vi "ziImpedance.vi"(9 "Eq Model":T1, 10 "Z (Ohm)":cdb[](array[numeric]) format="%_5p", 11 "Frequency (Hz)":dbl[](array[numeric]) format="%_6p") -> (2 "Labels and Units":string[][](array[string]), 3 "Values":dbl[][](array[numeric]))   [LabVIEW 2009, in "Zurich Instruments LabOne.lvlib"]
doc: "Calculate effective resistance, admittance and equivalen R||C circuit parameters for a DUT measured with an HF2 and an HF2CA.\n\n<B>Stimulation Amplitude (V)</B> (complex) in 4-point mode is the complex voltage amplitude measured accross the DUT (the user needs to account for Vrms to Vamplitude conversion by multiplying with sqrt(2)), in 2-point mode is the voltage amplitude applied to the DUT.\n<B>Measured (Vrms)</B> (complex) the measurement from HF2Camp.\n<B>Rci, Cci</B> Parasitic impedance between Z and preamp to gnd."
uses:
  <instrlib>/Zurich Instruments LabOne/Zurich Instruments LabOne.lvlib
  <instrlib>/Zurich Instruments LabOne/Public/Utility/Impedance/ziTypeImpedanceEqCircModel.ctl
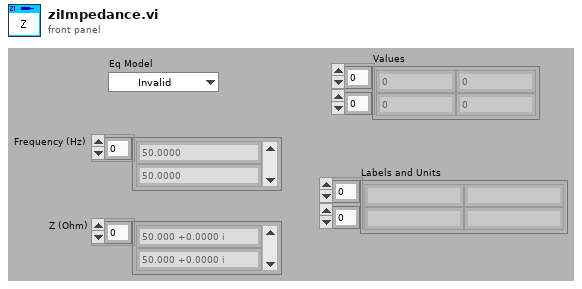
[diagram p1: front panel]
types:
  T1 = typedef "Zurich Instruments LabOne.lvlib/ziTypeImpedanceEqCircModel.ctl" = enum16{"Invalid", "|Z|, Phi", "R||C", "R||L", "R*C", "D*C", "R*L", "ReZ, ImZ", "G, B"}
  T2 = cluster{"label1":string, "label 2":string, "unit1":string, "unit2":string}[]
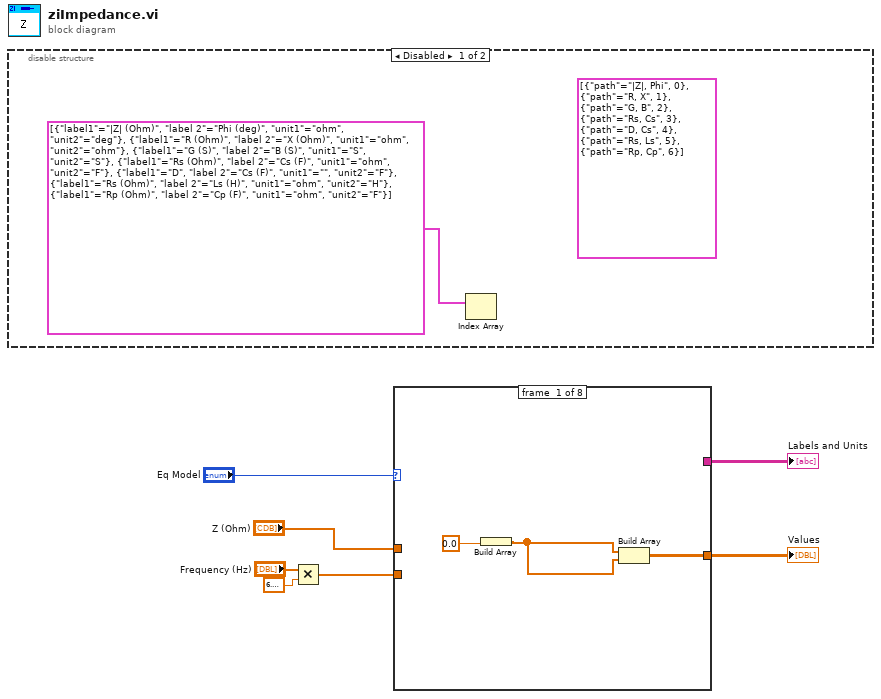
[diagram p0: block diagram]
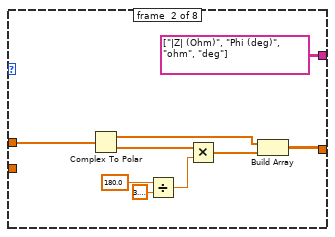
[diagram p3: hidden frame]
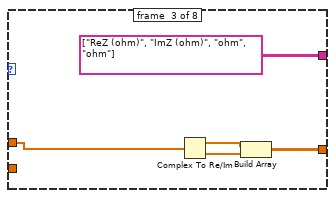
[diagram p4: hidden frame]
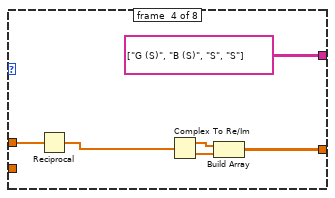
[diagram p5: hidden frame]
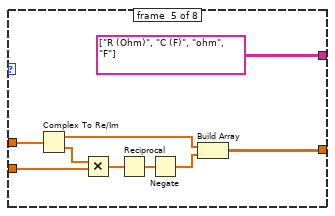
[diagram p6: hidden frame]
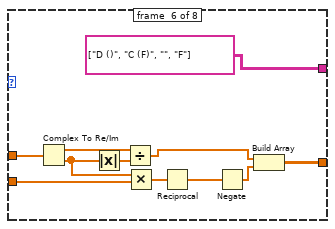
[diagram p7: hidden frame]
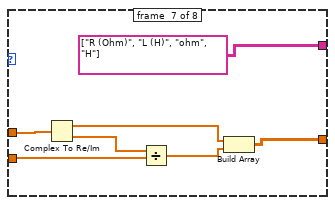
[diagram p8: hidden frame]
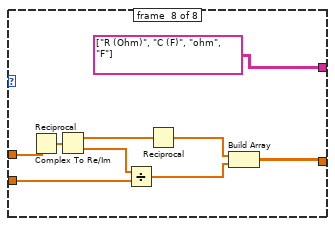
[diagram p9: hidden frame]
diagram:
  n1 = disable-structure shown="Disabled" {
    frame #0 {
      (unwired) cluster{"path":string, i32}[] [{"path"="|Z|, Phi", 0}, {"path"="R, X", 1}, {"path"="G, B", 2}, {"path"="Rs, Cs", 3}, {"path"="D, Cs", 4}, {"path"="Rs, Ls", 5}, {"path"="Rp, Cp", 6}]
      n2 = Index Array(array=T2 [{"label1"="|Z| (Ohm)", "label 2"="Phi (deg)", "unit1"="ohm", "unit2"="deg"}, {"label1"="R (Ohm)", "label 2"="X (Ohm)", "unit1"="ohm", "unit2"="ohm"}, {"label1"="G (S)", "label 2"="B (S)", "unit1"="S", "unit2"="S"}, {"label1"="Rs (Ohm)", "label 2"="Cs (F)", "unit1"="ohm", "unit2"="F"}, {"label1"="D", "label 2"="Cs (F)", "unit1"="", "unit2"="F"}, {"label1"="Rs (Ohm)", "label 2"="Ls (H)", "unit1"="ohm", "unit2"="H"}, {"label1"="Rp (Ohm)", "label 2"="Cp (F)", "unit1"="ohm", "unit2"="F"}]) -> ()  [unwired: 1 in, 1 out]
    }
    frame #1 {
    }
  }
  n3 = Multiply(x="Frequency (Hz)", y=6.283185307179586) -> (x*y=w5:dbl[])
  n4 = case shown="\"ReZ, ImZ\"" "Eq Model" {
    tunnel: w5 -> [_ _ _ _ w37 w49 w58 w64]
    tunnel: "Z (Ohm)" -> [_ w20 w25 w31 w40 w51 w57 w67]
    tunnel: [_ string[][] [["|Z| (Ohm)", "Phi (deg)"], ["ohm", "deg"]] string[][] [["ReZ (ohm)", "ImZ (ohm)"], ["ohm", "ohm"]] string[][] [["G (S)", "B (S)"], ["S", "S"]] string[][] [["R (Ohm)", "C (F)"], ["ohm", "F"]] string[][] [["D ()", "C (F)"], ["", "F"]] string[][] [["R (Ohm)", "L (H)"], ["ohm", "H"]] string[][] [["R (Ohm)", "C (F)"], ["ohm", "F"]]] -> w2
    tunnel: [w9 w12 w22 w27 w33 w42 w53 w60] -> w1
    frame #0 {
      n5 = Build Array(0.0) -> (w10:dbl[])
      n6 = Build Array(w10, w10) -> (w9:dbl[][])
    }
    frame #1 {
      n7 = Complex To Polar(r * e^(i*theta)=w20) -> (r=w14:dbl[], theta=w16:dbl[])
      n8 = Divide(x=180.0 ("y"), y=3.141592653589793) -> (x/y=w17:dbl)
      n9 = Multiply(x=w16, y=w17) -> (x*y=w13:dbl[])
      n10 = Build Array(w14, w13) -> (w12:dbl[][])
    }
    frame #2 {
      n11 = Complex To Re/Im(x + iy=w25) -> (x=w24:dbl[], y=w23:dbl[])
      n12 = Build Array(w24, w23) -> (w22:dbl[][])
    }
    frame #3 {
      n13 = Reciprocal(x=w31) -> (1/x=w30:cdb[])
      n14 = Complex To Re/Im(x + iy=w30) -> (x=w28:dbl[], y=w29:dbl[])
      n15 = Build Array(w28, w29) -> (w27:dbl[][])
    }
    frame #4 {
      n16 = Complex To Re/Im(x + iy=w40) -> (x=w35:dbl[], y=w38:dbl[])
      n17 = Multiply(x=w38, y=w37) -> (x*y=w39:dbl[])
      n18 = Reciprocal(x=w39) -> (1/x=w36:dbl[])
      n19 = Negate(x=w36) -> (-x=w34:dbl[])
      n20 = Build Array(w35, w34) -> (w33:dbl[][])
    }
    frame #5 {
      n21 = Complex To Re/Im(x + iy=w51) -> (x=w45:dbl[], y=w47:dbl[])
      n22 = Absolute Value(x=w47) -> (abs(x)=w46:dbl[])
      n23 = Divide(x=w45, y=w46) -> (x/y=w44:dbl[])
      n24 = Multiply(x=w47, y=w49) -> (x*y=w50:dbl[])
      n25 = Reciprocal(x=w50) -> (1/x=w48:dbl[])
      n26 = Negate(x=w48) -> (-x=w43:dbl[])
      n27 = Build Array(w44, w43) -> (w42:dbl[][])
    }
    frame #6 {
      n28 = Complex To Re/Im(x + iy=w57) -> (x=w55:dbl[], y=w56:dbl[])
      n29 = Divide(x=w56, y=w58) -> (x/y=w54:dbl[])
      n30 = Build Array(w55, w54) -> (w53:dbl[][])
    }
    frame #7 {
      n31 = Reciprocal(x=w67) -> (1/x=w66:cdb[])
      n32 = Complex To Re/Im(x + iy=w66) -> (x=w65:dbl[], y=w63:dbl[])
      n33 = Divide(x=w63, y=w64) -> (x/y=w61:dbl[])
      n34 = Reciprocal(x=w65) -> (1/x=w62:dbl[])
      n35 = Build Array(w62, w61) -> (w60:dbl[][])
    }
  }
  "Labels and Units" <- w2
  "Values" <- w1
